vi "BRig_RT_loadData__subunit1.vi"(10 "input_data":u16[](array[numeric]), 11 "input_name":string="dataExp") -> (2 "output_data":u16[](array[numeric]))   [LabVIEW 2014]
uses:
  <vilib>/Utility/file.llb/Read From Spreadsheet File (I64).vi
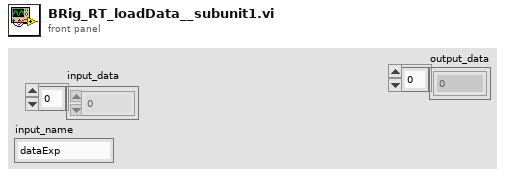
[diagram p1: front panel]
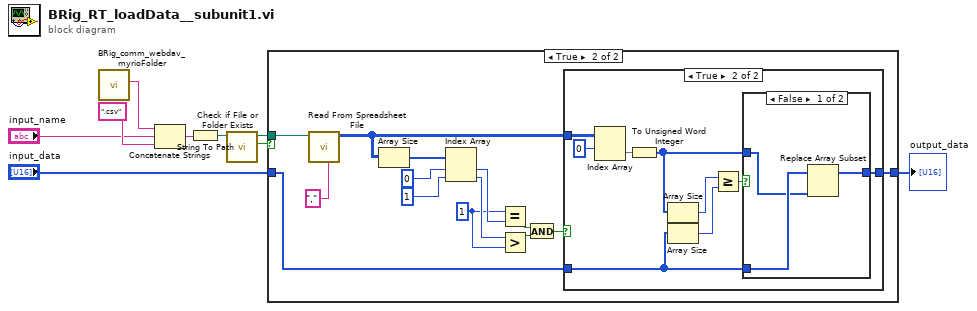
[diagram p0: block diagram]
diagram:
  n1 = call "BRig_comm_webdav_myrioFolder.vi"() -> ("output_myrioFolder"=w9:string)  [unwired: 11 in]
  n2 = Concatenate Strings(w9, "input_name", ".csv" ("string")) -> (w7:string)
  n3 = String To Path(string=w7) -> (path=w5:path)
  n4 = call <vilib>:"Check if File or Folder Exists.vi"("path"=w5) -> ("file or folder exists?"=w4:bool, "dup path"=w3:path)  [unwired: 8 in, 1 out]
  n5 = case shown="True" w4 {
    tunnel: w3 -> [_ w24]
    tunnel: "input_data" -> [w10 w18]
    tunnel: [w10 w17] -> w1
    frame False {
    }
    frame True {
      w12 = 1 ("x")
      n6 = call-poly <vilib>:"Read From Spreadsheet File.vi"("delimiter (\\t)"="," ("delimiter (\\t)"), "file path (dialog if empty)"=w24) -> ("all rows"=w16:i64[][])  [unwired: 5 in, 4 out]
      n7 = Array Size(array=w16) -> (size(s)=w22:i32[])
      n8 = Index Array(array=w22, index #1=0 ("index"), index #2=1 ("index")) -> (element #1=w15:i32, element #2=w13:i32)
      n9 = Equal?(x=w12, y=w15) -> (x = y?=w14:bool)
      n10 = Greater?(x=w13, y=w12) -> (0:w11:bool)
      n11 = And(x=w14, y=w11) -> (x .and. y?=w19:bool)
      n12 = case shown="True" w19 {
        tunnel: w18 -> [w25 w26]
        tunnel: [w25 w27] -> w17
        tunnel: w16 -> [_ w34]
        frame False {
        }
        frame True {
          n13 = Index Array(array=w34, index (row)=0) -> (element=w32:i64[])  [unwired: 1 in]
          n14 = To Unsigned Word Integer(number=w32) -> (unsigned 16bit integer=w28:u16[])
          n15 = Array Size(array=w28) -> (size(s)=w31:i32)
          n16 = Array Size(array=w26) -> (size(s)=w30:i32)
          n17 = Greater Or Equal?(x=w31, y=w30) -> (x >= y?=w29:bool)
          n18 = case shown="False" w29 {
            tunnel: w28 -> [w36 w38]
            tunnel: [w35 w38] -> w27
            tunnel: w26 -> [w37 _]
            frame False {
              n19 = Replace Array Subset(array=w37, new element=w36) -> (w35:u16[])  [unwired: 1 in]
            }
            frame True {
            }
          }
        }
      }
    }
  }
  "output_data" <- w1
